vi "QuVI_Wire.vi"   [LabVIEW 2020]
doc: "Initializes a qubit in the state |0> and provides a reference wire for circuit construction.\n\nThis VI serves as the fundamental starting point for any quantum circuit in the QuVI toolkit. It effectively initializes a single qubit in the ground state |0>.\n\nTo build a multi-qubit register, stack multiple instances of this VI vertically on the block diagram. The vertical connections aggregate the qubit count for the global state vector.\n\nTerminals:\n\n[Top] Stack in: Connect from the 'Stack out' of the previous qubit above. Leave unconnected for the first qubit (Qubit 0).\n\n[Bottom] Stack out: Connect to the 'Stack in' of the next qubit below.\n\n[Right] Quantum Wire Ref: The \"QuWire.\" Connect this to the left border of a Flat Sequence Structure."
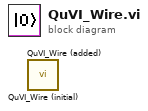
[diagram p0: block diagram]
diagram:
  n1 = call "QuVI_Wire (initial).vi"() -> ()  [unwired: 14 in, 2 out]
  n2 = call "QuVI_Wire (added).vi"() -> ()  [unwired: 14 in, 2 out]
